vi "Last Ack Creator.vi"(10 "jettl":refnum<class "jettl.lvclass">) -> (2 "Msg Strategy":refnum<class "Msg Strategy.lvclass">)   [LabVIEW 2021, in "jettl.lvlib" / "Last Ack Creator Msg Strategy.lvlib"]
uses:
  Last Ack Creator Msg Strategy.lvlib
  Last Ack Creator Msg Strategy/Last Ack Creator Msg Strategy.lvclass
  C:/git/jettl/jettl/jettl/Last Ack Creator Msg Strategy/Last Ack Creator Msg Strategy/Last Ack Creator Msg Strategy.lvclass
  C:/git/jettl/jettl/jettl/Msg Strategy/Msg Strategy.lvclass
  Msg Strategy/Msg Strategy.lvclass
  jettl/jettl.lvclass
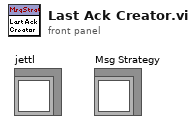
[diagram p1: front panel]
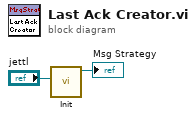
[diagram p0: block diagram]
diagram:
  n1 = call "Init.vi"("jettl"="jettl") -> ("Last Ack Creator Msg Strategy out"=→"Msg Strategy":refnum<class "Last Ack Creator Msg Strategy.lvclass">)  [unwired: 10 in]
